vi "PostCopyScripting (bkup).vi"(10 "MetaDataObj":refnum<class "MetaDataObj.lvclass">, 11 "User Project":refnum<vi>) -> ()   [LabVIEW 2013]
uses:
  <resource>/dialog/NewProjectWizard/MetaDataObj/MetaDataObj.lvclass
  FixedChannelTBModuleDecideFeatures.lvclass
  FixedChannelTBModuleDecideFeatures.lvclass/FixedChannelTBModuleDecideFeatures.ctl
  Read component name.vi
  Read Channel Specification.vi
  <resource>/dialog/NewProjectWizard/MetaDataObj/Accessors/Read Project Path.vi
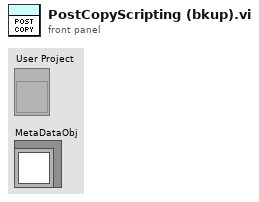
[diagram p1: front panel]
types:
  T1 = typedef "channel configuration.ctl" = cluster{"Name":string, "channel classification":T2, "data type":T3}
  T2 = typedef "TBM channel.lvclass/channel classification.ctl" = enum16{"input data", "output data", "processing parameter", "processing result"}
  T3 = typedef "tag bus.lvlib/tag descriptor.lvclass/Data Type.ctl" = enum16{"Double", "Single", "I64", "I32", "I16", "I8", "U64", "U32", "U16", "U8", "Boolean", "String", "Array of Double", "Array of Single", "Array of I64", "Array of I32", "Array of I16", "Array of I8", "Array of U64", "Array of U32", "Array of U16", "Array of U8", "Array of Boolean", "Array of String"}
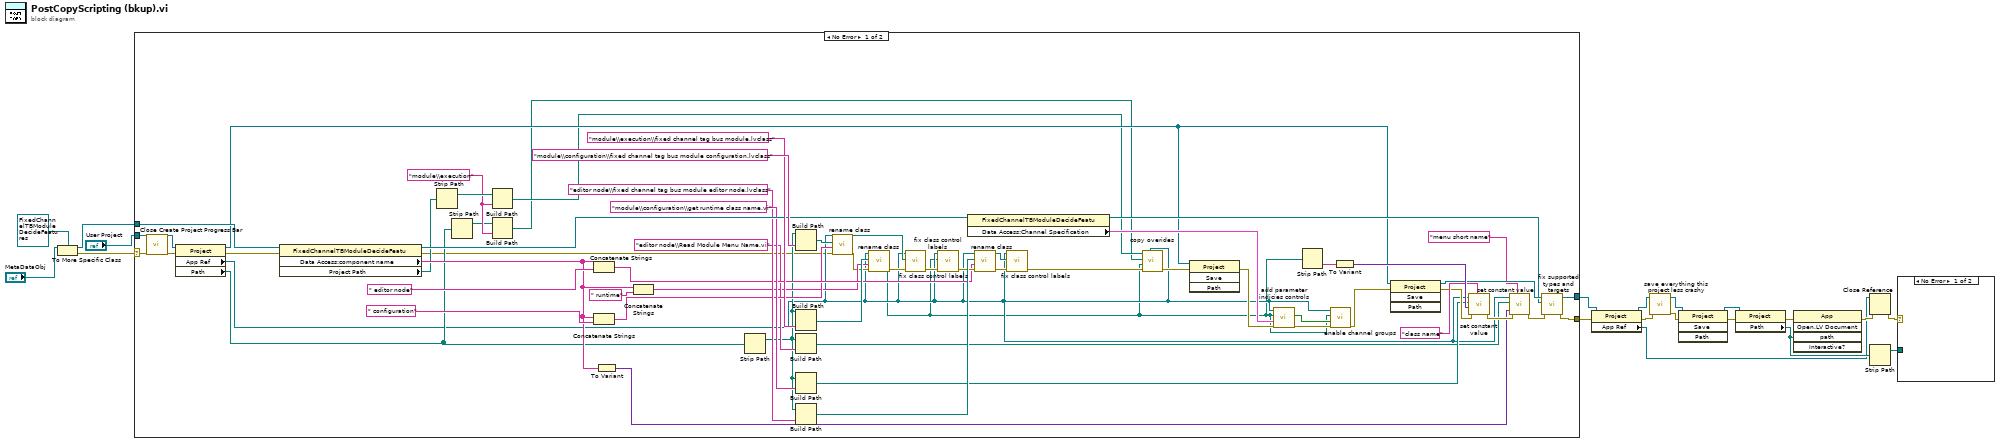
[diagram p0: block diagram]
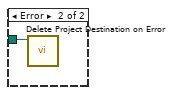
[diagram p2: hidden frame]
diagram:
  n1 = To More Specific Class(target class=refnum<class "FixedChannelTBModuleDecideFeatures.lvclass"> refnum ("DecideProjectFeatures.lvclass"), reference="MetaDataObj") -> (specific class reference=w10:refnum<class "FixedChannelTBModuleDecideFeatures.lvclass">, error out=w17:errorcluster)  [unwired: 1 in]
  n2 = case shown="No Error" w17 {
    selector: w17 -> [w68 w82]
    tunnel: [w56 w83] -> w8
    tunnel: "User Project" -> [w67 w83]
    tunnel: [w57 w82] -> w7
    tunnel: w10 -> [w79 _]
    frame No Error {
      w31 = "module\\execution"
      n3 = call <resource>:"Close Create Project Progress Bar.vi"("error in (no error)"=w68, "Project"=w67) -> ("error out"=w65:errorcluster, "dup Project"=w66:refnum<vi>)  [unwired: 8 in]
      n4 = property class="Project"(reference=w66, error in=w65) -> (reference out=w34:refnum<vi>, error out=w26:errorcluster, "App Ref"=w22:refnum<vi>, "Path"=w29:path)
      n5 = property class="FixedChannelTBModuleDecideFeatu"(reference=w79, error in=w26) -> (reference out=w76:refnum<class "FixedChannelTBModuleDecideFeatures.lvclass">, error out=w20:errorcluster, "Data Access:component name"=w43:string, "Project Path"=w33:path)
      n6 = Strip Path(path=w33) -> (stripped path=w32:path)  [unwired: 1 out]
      n7 = Strip Path(path=w29) -> (stripped path=w28:path)  [unwired: 1 out]
      n8 = Build Path(base path=w32, name or relative path=w31) -> (appended path=w30:path)
      n9 = Build Path(base path=w28, name or relative path=w31) -> (appended path=w25:path)
      n10 = Concatenate Strings(w43, " editor node" ("string")) -> (w58:string)
      n11 = Concatenate Strings(w43, " configuration" ("string")) -> (w54:string)
      n12 = To Variant(anything=w43) -> (Variant=w49:variant)
      n13 = Concatenate Strings(w43, " runtime" ("string")) -> (w45:string)
      n14 = Strip Path(path=w29) -> (stripped path=w44:path)  [unwired: 1 out]
      n15 = Build Path(base path=w44, name or relative path="module\\configuration\\fixed channel tag bus module configuration.lvclass") -> (appended path=w41:path)
      n16 = Build Path(base path=w44, name or relative path="module\\execution\\fixed channel tag bus module.lvclass") -> (appended path=w78:path)
      n17 = Build Path(base path=w44, name or relative path="editor node\\Read Module Menu Name.vi") -> (appended path=w47:path)
      n18 = Build Path(base path=w44, name or relative path="module\\configuration\\get runtime class name.vi") -> (appended path=w53:path)
      n19 = Build Path(base path=w44, name or relative path="editor node\\fixed channel tag bus module editor node.lvclass") -> (appended path=w63:path)
      n20 = call "rename class.vi"("error in"=w20, "new name"=w54, "class path"=w41, "Application in"=w22) -> ("error out"=w42:errorcluster, "New Library Path"=w40:path)  [unwired: 6 in]
      n21 = call "rename class.vi"("error in"=w42, "new name"=w45, "class path"=w78, "Application in"=w22) -> ("error out"=w70:errorcluster, "New Library Path"=w21:path)  [unwired: 6 in]
      n22 = call "fix class control labels.vi"("error in"=w70, "class to load"=w40, "Application in"=w22) -> ("error out"=w69:errorcluster)  [unwired: 8 in]
      n23 = call "fix class control labels.vi"("error in"=w69, "class to load"=w21, "Application in"=w22) -> ("error out"=w60:errorcluster)  [unwired: 8 in]
      n24 = property class="FixedChannelTBModuleDecideFeatu"(reference=w76) -> (reference out=w39:refnum<class "FixedChannelTBModuleDecideFeatures.lvclass">, "Data Access:Channel Specification"=w38:T1[])  [unwired: 1 in, 1 out]
      n25 = call "rename class.vi"("error in"=w60, "new name"=w58, "class path"=w63, "Application in"=w22) -> ("error out"=w61:errorcluster, "New Library Path"=w62:path)  [unwired: 6 in]
      n26 = call "fix class control labels.vi"("error in"=w61, "class to load"=w62, "Application in"=w22) -> ("error out"=w23:errorcluster)  [unwired: 8 in]
      n27 = call "copy overides.vi"("application reference (local)"=w22, "error in"=w23, "New class path"=w21, "New path"=w25, "Old Path"=w30) -> ("error out"=w24:errorcluster)  [unwired: 6 in]
      n28 = invoke class="Project" method="Save"(reference=w34, error in=w24) -> (error out=w37:errorcluster)  [unwired: 2 in, 3 out]
      n29 = call "add parameter indicies controls.vi"("error in"=w37, "Channels to create"=w38, "class path"=w21, "Application in"=w22) -> ("error out"=w36:errorcluster, "Disable Channel Group?"=w35:bool[])  [unwired: 6 in]
      n30 = Strip Path(path=w21) -> (name=w52:string)  [unwired: 1 out]
      n31 = call "enable channel groups.vi"("error in"=w36, "Disable channel group?"=w35, "class path"=w21, "Application in"=w22) -> ("error out"=w27:errorcluster)  [unwired: 7 in]
      n32 = To Variant(anything=w52) -> (Variant=w75:variant)
      n33 = invoke class="Project" method="Save"(reference=w34, error in=w27) -> (reference out=w71:refnum<vi>, error out=w72:errorcluster)  [unwired: 2 in, 2 out]
      n34 = call "set constant value.vi"("control name"="class name", "error in"=w72, "data to set"=w75, "vi path"=w53, "Application in"=w22) -> ("error out"=w55:errorcluster)  [unwired: 6 in]
      n35 = call "set constant value.vi"("control name"="menu short name", "error in"=w55, "data to set"=w49, "vi path"=w47, "Application in"=w22) -> ("error out"=w51:errorcluster)  [unwired: 6 in]
      n36 = call "fix supported types and targets.vi"("error in"=w51, "DecideProjectFeatures in"=w39, "User Project in"=w71) -> ("error out"=w57:errorcluster, "User Project out"=w56:refnum<vi>)  [unwired: 7 in]
    }
    frame Error {
    }
  }
  n37 = property class="Project"(reference=w8, error in=w7) -> (reference out=w5:refnum<vi>, error out=w6:errorcluster, "App Ref"=w4:refnum<vi>)
  n38 = call "save everything this project less crashy.vi"("error in"=w6, "Project in"=w5) -> ("error out"=w1:errorcluster, "Project out"=w9:refnum<vi>)  [unwired: 8 in]
  n39 = invoke class="Project" method="Save"(reference=w9, error in=w1) -> (reference out=w13:refnum<vi>, error out=w14:errorcluster)  [unwired: 2 in, 2 out]
  n40 = property class="Project"(reference=w13, error in=w14) -> (error out=w16:errorcluster, "Path"=w11:path)  [unwired: 1 out]
  n41 = invoke class="App" method="Open.LV Document"(error in=w16, "path"=w11) -> (error out=w15:errorcluster)  [unwired: 3 in, 4 out]
  n42 = Close Reference(reference=w4, error in (no error)=w15) -> (error out=w3:errorcluster)
  n43 = Strip Path(path=w11) -> (stripped path=w2:path)  [unwired: 1 out]
  n44 = case shown="No Error" w3 {
    tunnel: w2 -> [_ w84]
    frame No Error {
    }
    frame Error {
      n45 = call <resource>:"Delete Project Destination on Error.vi"("Project Destination Root"=w84) -> ()  [unwired: 11 in]
    }
  }
